vi "SS2 Live_Live Image Message.vi"(6 "Init":bool, 8 "error in (no error)":errorcluster, 11 "SS2 Live Internal Variables":T3={"okCFrontPanelDevices Refnum"=refnum, "Device Refnum"=refnum, "Display Image"=refnum, "# Live Images"=0, "relative s"=0.0, "# Image Sets"=0, "Message"="", "Current Image Set"=0, "# Datasets"=0, "Current Dataset"=0, "Live Mode"=FALSE, "Recording Mode"=FALSE, "Record Button"=refnum, "Live Button"=refnum, "SS2 Live Gate Data Q Name"="SS2 Live Gate Data Q", "Discard First Image"=FALSE, "Image Information"={"Save ROI Only"=FALSE, "Left"=0, "Top"=0, "Right"=0, "Bottom"=0, "Use Current ROI"=FALSE}, "Image Binning Options"={"Use Image Binning"=FALSE, "X Bin"=1, "Y Bin"=1}, "FPGA Serial Number"="", "PCB Version"=enum."PCB 1"} {"Image Binning Options"."Y Bin" min=1; "Image Binning Options"."X Bin" min=1}) -> (0 "error out":errorcluster, 1 "Message":string, 2 "SS2 Live Atomic Action":T1={"SS2 Q Event"=enum."Idle", "Data"=variant}, 3 "SS2 Live Internal Variables":T3={"okCFrontPanelDevices Refnum"=refnum, "Device Refnum"=refnum, "Display Image"=refnum, "# Live Images"=0, "relative s"=0.0, "# Image Sets"=0, "Message"="", "Current Image Set"=0, "# Datasets"=0, "Current Dataset"=0, "Live Mode"=FALSE, "Recording Mode"=FALSE, "Record Button"=refnum, "Live Button"=refnum, "SS2 Live Gate Data Q Name"="SS2 Live Gate Data Q", "Discard First Image"=FALSE, "Image Information"={"Save ROI Only"=FALSE, "Left"=0, "Top"=0, "Right"=0, "Bottom"=0, "Use Current ROI"=FALSE}, "Image Binning Options"={"Use Image Binning"=FALSE, "X Bin"=1, "Y Bin"=1}, "FPGA Serial Number"="", "PCB Version"=enum."PCB 1"} {"Image Binning Options"."Y Bin" min=1; "Image Binning Options"."X Bin" min=1})   [LabVIEW 2019]
uses:
  SS2 Live Internal Variables.ctl
  C:/UCLA Thinkpad Google Drive/LabVIEW 2019 SP1/builds/SS2 Live Distribution/Opal Kelly/C# Wrapper/libFrontPanel-csharp.dll
  Opal Kelly/C# Wrapper/libFrontPanel-csharp.dll
  <vilib>/vision/Image Controls.llb/IMAQ Image.ctl
  SS2 Live_Image ROI Information.ctl
  Phasor/Image Binning Options.ctl
  SS2 DAQ PCB Version.ctl
  SS2 Q [Element].ctl
  SS2 Q Event List.ctl
  <vilib>/Utility/High Resolution Relative Seconds.vi
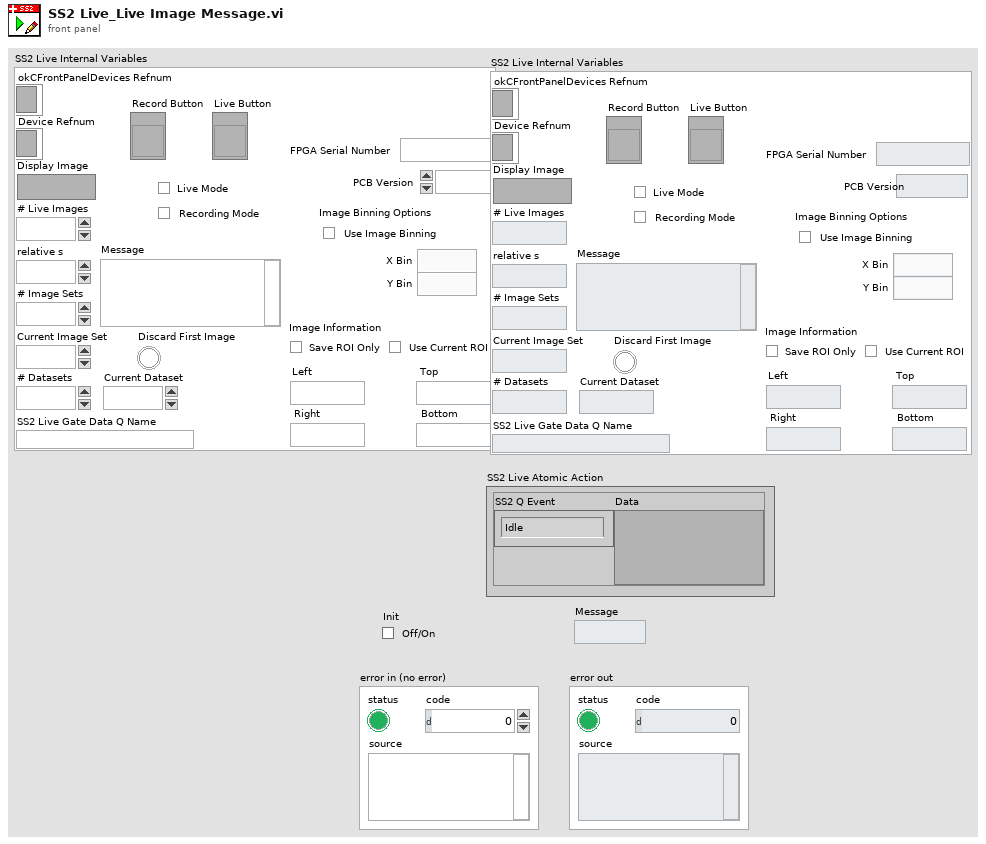
[diagram p1: front panel]
types:
  T1 = typedef "SS2 Q [Element].ctl" = cluster{"SS2 Q Event":T2, "Data":variant}
  T2 = typedef "SS2 Q Event List.ctl" = enum16{"---- UI ----", "Idle", "Initialization", "FPGA Status", "Reset FPGA", "Quit", "---- DAQ ----", "Start Recording", "Start Live Acquisition", "Initialize Recording Mode", "Initialize FPGA (Live Mode)", "Get Image Set", "Get Single Image", "Update Image Display", "Stop Live Acquisition", "Stop Data Recording", "Stop Data Saving", "---- Image ----", "Copy Data to Clipboard", "Set Image Palette", "Save Displayed Image with Overlay", "Save Image Data as TIFF"}
  T3 = typedef "SS2 Live Internal Variables.ctl" = cluster{"okCFrontPanelDevices Refnum":refnum<k24>, "Device Refnum":refnum<k24>, "Display Image":T4, "# Live Images":i32, "relative s":dbl, "# Image Sets":i32, "Message":string, "Current Image Set":i32, "# Datasets":i32, "Current Dataset":i32, "Live Mode":bool, "Recording Mode":bool, "Record Button":refnum<vi>, "Live Button":refnum<vi>, "SS2 Live Gate Data Q Name":string, "Discard First Image":bool, "Image Information":T5, "Image Binning Options":T6, "FPGA Serial Number":string, "PCB Version":T7}
  T4 = typedef "IMAQ Image.ctl" = refnum<image>
  T5 = typedef "SS2 Live_Image ROI Information.ctl" = cluster{"Save ROI Only":bool, "Left":u16, "Top":u16, "Right":u16, "Bottom":u16, "Use Current ROI":bool}
  T6 = typedef "Image Binning Options.ctl" = cluster{"Use Image Binning":bool, "X Bin":i32, "Y Bin":i32}
  T7 = typedef "SS2 DAQ PCB Version.ctl" = enum16{"unknown", "PCB 1", "PCB 2"}
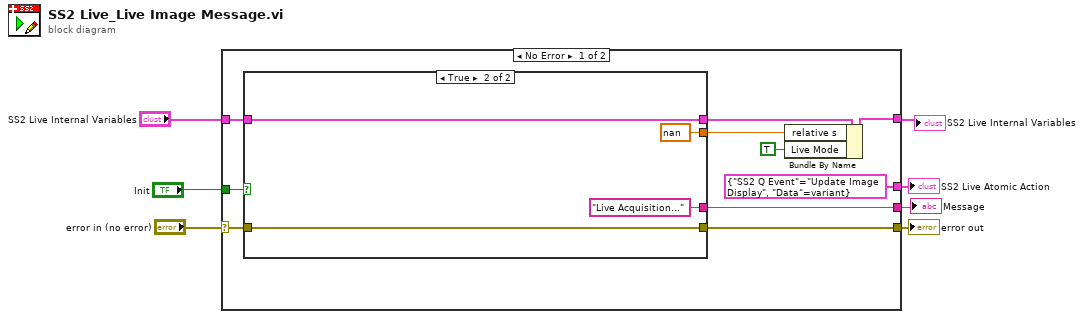
[diagram p0: block diagram]
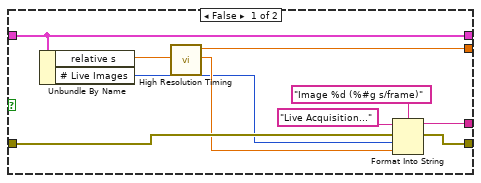
[diagram p2: hidden frame]
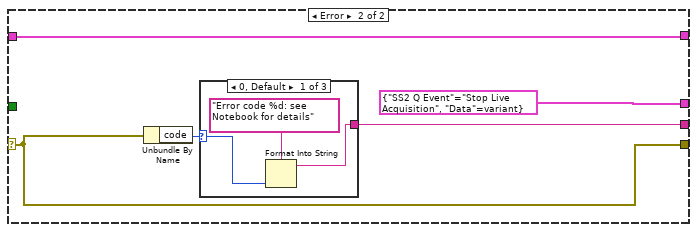
[diagram p3: hidden frame]
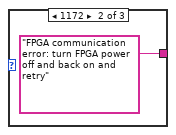
[diagram p4: hidden frame]
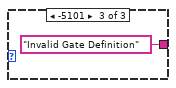
[diagram p5: hidden frame]
diagram:
  n1 = case shown="No Error" "error in (no error)" {
    selector: "error in (no error)" -> [w16 w34]
    tunnel: [w17 w34] -> w7
    tunnel: [w15 w35] -> w5
    tunnel: "SS2 Live Internal Variables" -> [w13 w33]
    tunnel: [w14 w33] -> w3
    tunnel: "Init" -> [w11 _]
    tunnel: [T1 {"SS2 Q Event"=enum."Update Image Display", "Data"=variant} ("SS2 Live Atomic Action") T1 {"SS2 Q Event"=enum."Stop Live Acquisition", "Data"=variant} ("SS2 Live Atomic Action")] -> w1
    frame No Error {
      n2 = case shown="True" w11 {
        tunnel: [w26 w28] -> w17
        tunnel: w16 -> [w25 w28]
        tunnel: [w24 "Live Acquisition..."] -> w15
        tunnel: w13 -> [w19 w29]
        tunnel: [w21 nan ("relative seconds")] -> w12
        tunnel: [w19 w29] -> w10
        frame False {
          n3 = Unbundle By Name(w19) -> ("relative s"=w22:dbl, "# Live Images"=w18:i32)
          n4 = call "High Resolution Timing.vi"("relative seconds (NaN)"=w22) -> ("relative seconds"=w21:dbl, "elapsed (relative) seconds"=w20:dbl)  [unwired: 16 in, 1 out]
          n5 = Format Into String(format string="Image %d (%#g s/frame)", initial string="Live Acquisition..." ("Message"), error in=w25, w18, w20) -> (resulting string=w24:string, error out=w26:errorcluster)
        }
        frame True {
        }
      }
      n6 = Bundle By Name(cluster=w10, "relative s"=w12, "Live Mode"=TRUE) -> (w14:T3)
    }
    frame Error {
      n7 = Unbundle By Name(w34) -> ("code"=w36:i32)
      n8 = case shown="0, Default" w36 {
        selector: w36 -> [w38 _ _]
        tunnel: [w39 "FPGA communication error: turn FPGA power off and back on and retry" "Invalid Gate Definition"] -> w35
        frame 0, Default {
          n9 = Format Into String(format string="Error code %d: see Notebook for details", w38) -> (resulting string=w39:string)  [unwired: 2 in, 1 out]
        }
        frame 1172 {
        }
        frame -5101 {
        }
      }
    }
  }
  "error out" <- w7
  "Message" <- w5
  "SS2 Live Internal Variables" <- w3
  "SS2 Live Atomic Action" <- w1
